vi "pLogicEngine.vi"(8 "error in":errorcluster, 9 "Sequence":string[][](array[string]), 10 "data dictionary in":refnum<class "data dictionary.lvclass">, 11 "default data table":T1) -> (0 "error out":errorcluster, 3 "data table out":T1)   [LabVIEW 2013]
uses:
  <vilib>/NI/Tag Bus/table/data table.ctl
  <vilib>/NI/Tag Bus/dictionary/data dictionary.lvclass
  Controls/RungLogicState.ctl
  <vilib>/NI/Tag Bus/tag/Data Type.ctl
  <vilib>/NI/Tag Bus/table/data polymorphs/read one/read Boolean.vi
  <vilib>/NI/Tag Bus/table/data polymorphs/write one/write Boolean.vi
  <vilib>/NI/Tag Bus/tag/tag descriptor.lvclass
  <vilib>/NI/Tag Bus/table/data table.lvlib
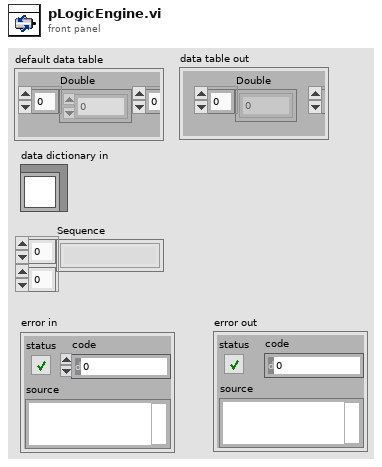
[diagram p1: front panel]
types:
  T1 = typedef "tag bus.lvlib/data table.lvlib/data table.ctl" = cluster{"Double":dbl[], "Single":sgl[], "I64":i64[], "I32":i32[], "I16":i16[], "I8":i8[], "U64":u64[], "U32":u32[], "U16":u16[], "U8":u8[], "Boolean":bool[], "String":string[], "Array of Double":cluster{"DBL Array":dbl[]}[], "Array of Single":cluster{"SGL Array":sgl[]}[], "Array of I64":cluster{"I64 Array":i64[]}[], "Array of I32":cluster{"I32 Array":i32[]}[], "Array of I16":cluster{"I16 Array":i16[]}[], "Array of I8":cluster{"I8 Array":i8[]}[], "Array of U64":cluster{"U64 Array":u64[]}[], "Array of U32":cluster{"U32 Array":u32[]}[], "Array of U16":cluster{"U16 Array":u16[]}[], "Array of U8":cluster{"U8 Array":u8[]}[], "Array of Boolean":cluster{"Boolean Array":bool[]}[], "Array of String":cluster{"String Array":string[]}[]}
  T2 = typedef "RungLogicState.ctl" = cluster{"Rung State":bool, "prev value":bool, "prev index":i32}
  T3 = typedef "tag bus.lvlib/tag descriptor.lvclass/Data Type.ctl" = enum16{"Double", "Single", "I64", "I32", "I16", "I8", "U64", "U32", "U16", "U8", "Boolean", "String", "Array of Double", "Array of Single", "Array of I64", "Array of I32", "Array of I16", "Array of I8", "Array of U64", "Array of U32", "Array of U16", "Array of U8", "Array of Boolean", "Array of String"}
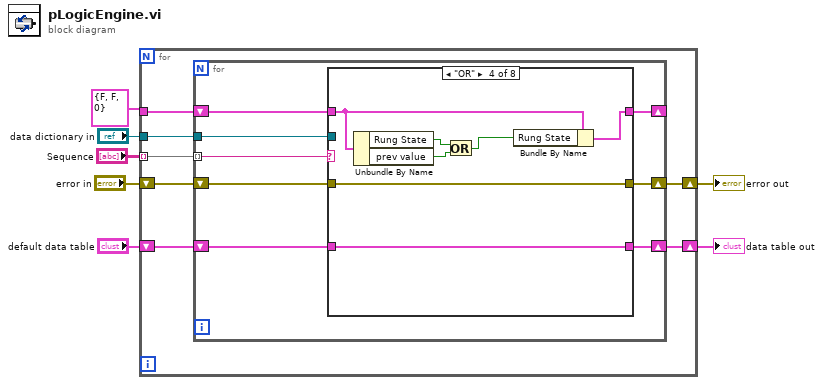
[diagram p0: block diagram]
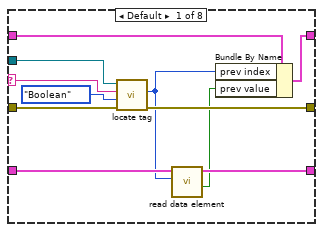
[diagram p2: hidden frame]
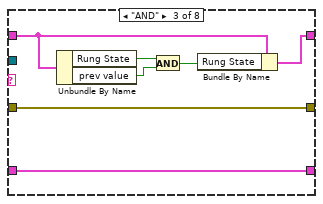
[diagram p4: hidden frame]
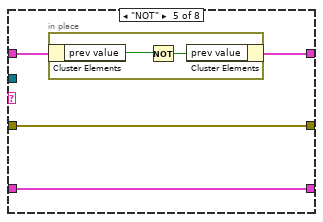
[diagram p5: hidden frame]
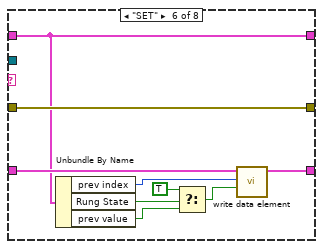
[diagram p6: hidden frame]
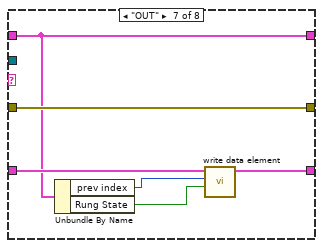
[diagram p7: hidden frame]
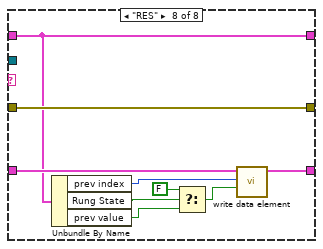
[diagram p8: hidden frame]
diagram:
  n1 = for {
    tunnel: "Sequence" -> [w14] mode=indexing
    tunnel: "data dictionary in" -> [w11]
    shift-right: [w12] -> w5
    shift-left: "default data table" -> [w13]
    shift-right: [w9] -> w7
    shift-left: "error in" -> [w10]
    tunnel: T2 {"Rung State"=FALSE, "prev value"=FALSE, "prev index"=0} -> [w8]
    n2 = for {
      tunnel: w14 -> [w22] mode=indexing
      tunnel: w11 -> [w21]
      shift-right: [w19] -> w12
      shift-left: w13 -> [w20]
      shift-right: [w17] -> w9
      shift-left: w10 -> [w18]
      shift-right: [w16] -> _
      shift-left: w8 -> [w15]
      n3 = case shown="\"OR\"" w22 {
        selector: w22 -> [w31 _ _ _ _ _ _ _]
        tunnel: w21 -> [w32 _ _ _ _ _ _ _]
        tunnel: w20 -> [w33 w36 w43 w50 w54 w62 w70 w77]
        tunnel: [w29 w36 w43 w50 w54 w65 w71 w80] -> w19
        tunnel: w18 -> [w28 w35 w42 w49 w53 w61 w69 w76]
        tunnel: [w27 w35 w42 w49 w53 w61 w69 w76] -> w17
        tunnel: [w23 w34 w40 w47 w51 w60 w68 w75] -> w16
        tunnel: w15 -> [w26 w34 w41 w48 w52 w60 w68 w75]
        frame Default {
          n4 = call <vilib>:"locate tag.vi"("error in"=w28, "data type"=Data_Type."Boolean", "name"=w31, "data dictionary in"=w32) -> ("error out"=w27:errorcluster, "index"=w25:i32)  [unwired: 5 in, 1 out]
          n5 = call-poly <vilib>:"read data element.vi"("index"=w25, "data table in"=w33) -> ("value"=w24:bool, "data table out"=w29:T1)  [unwired: 8 in]
          n6 = Bundle By Name(cluster=w26, "prev index"=w25, "prev value"=w24) -> (w23:T2)
        }
        frame "" {
        }
        frame "AND" {
          n7 = Unbundle By Name(w41) -> ("Rung State"=w38:bool, "prev value"=w37:bool)
          n8 = And(x=w38, y=w37) -> (x .and. y?=w39:bool)
          n9 = Bundle By Name(cluster=w41, "Rung State"=w39) -> (w40:T2)
        }
        frame "OR" {
          n10 = Unbundle By Name(w48) -> ("Rung State"=w46:bool, "prev value"=w45:bool)
          n11 = Or(x=w46, y=w45) -> (x .or. y?=w44:bool)
          n12 = Bundle By Name(cluster=w48, "Rung State"=w44) -> (w47:T2)
        }
        frame "NOT" {
          n13 = in-place {
            n14 = in-place-cluster #1(w52) -> ("prev value"=w56:bool)
            n15 = Not(x=w56) -> (.not. x?=w55:bool)
            n16 = in-place-cluster #1("prev value"=w55) -> (w51:T2)
          }
        }
        frame "SET" {
          n17 = Unbundle By Name(w60) -> ("prev index"=w57:i32, "Rung State"=w59:bool, "prev value"=w58:bool)
          n18 = Select(t=TRUE, s=w59, f=w58) -> (s? t:f=w63:bool)
          n19 = call-poly <vilib>:"write data element.vi"("value"=w63, "index"=w57, "data table in"=w62) -> ("data table out"=w65:T1)  [unwired: 8 in]
        }
        frame "OUT" {
          n20 = Unbundle By Name(w68) -> ("prev index"=w66:i32, "Rung State"=w67:bool)
          n21 = call-poly <vilib>:"write data element.vi"("value"=w67, "index"=w66, "data table in"=w70) -> ("data table out"=w71:T1)  [unwired: 8 in]
        }
        frame "RES" {
          n22 = Unbundle By Name(w75) -> ("prev index"=w72:i32, "Rung State"=w73:bool, "prev value"=w74:bool)
          n23 = Select(t=FALSE, s=w73, f=w74) -> (s? t:f=w78:bool)
          n24 = call-poly <vilib>:"write data element.vi"("value"=w78, "index"=w72, "data table in"=w77) -> ("data table out"=w80:T1)  [unwired: 8 in]
        }
      }
    }
  }
  "error out" <- w7
  "data table out" <- w5
